vi "addCommand.vi"(8 "error in (no error)":errorcluster, 10 "Command.lvclass":refnum<class "Command.lvclass">, 11 "CommandQueue in":refnum<class "CommandQueue.lvclass">) -> (0 "error out":errorcluster, 3 "CommandQueue out":refnum<class "CommandQueue.lvclass">)   [LabVIEW 2020, in "CommandQueue.lvclass"]
uses:
  CommandQueue.lvclass
  Command/Command.lvclass
  CommandQueue.lvclass/CommandQueue.ctl
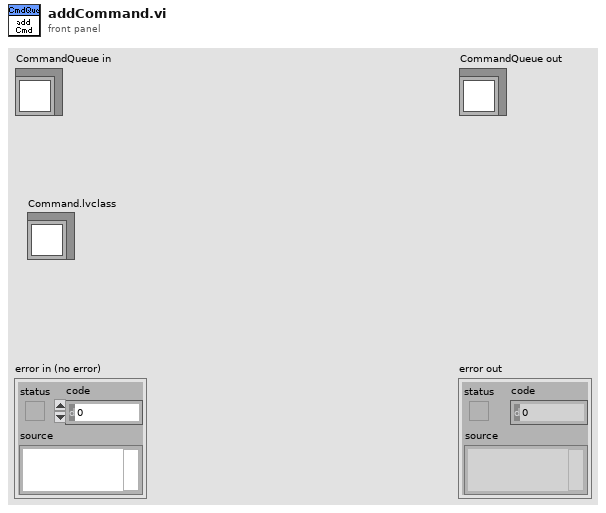
[diagram p1: front panel]
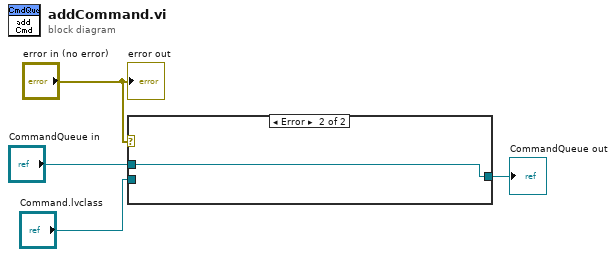
[diagram p0: block diagram]
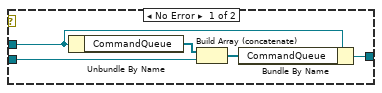
[diagram p2: hidden frame]
diagram:
  n1 = case shown="Error" "error in (no error)" {
    tunnel: "CommandQueue in" -> [w9 w10]
    tunnel: [w8 w10] -> w3
    tunnel: "Command.lvclass" -> [w6 _]
    frame No Error {
      n2 = Unbundle By Name(w9) -> ("CommandQueue"=w7:refnum<class "Command.lvclass">[])
      n3 = Build Array (concatenate)(w7, w6) -> (w5:refnum<class "Command.lvclass">[])
      n4 = Bundle By Name(cluster=w9, "CommandQueue"=w5) -> (w8:refnum<class "CommandQueue.lvclass">)
    }
    frame Error {
    }
  }
  "CommandQueue out" <- w3
  "error out" <- "error in (no error)"
